vi "GetLastTrue.vi"(8 "Default value":i32, 11 "Input":bool[](array[boolean])) -> (3 "Last True":i32)   [LabVIEW 2014]
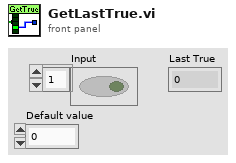
[diagram p1: front panel]
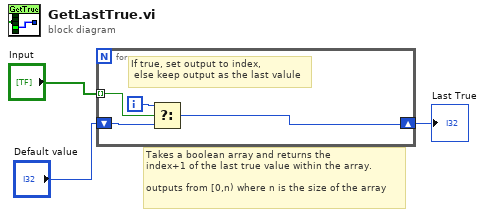
[diagram p0: block diagram]
diagram:
  # "Takes a boolean array and returns the \nindex+1 of the last true value within the array.\n\noutputs from [0,n) where n is the size of the array"
  n1 = for {
    tunnel: "Input" -> [w6] mode=indexing
    shift-right: [w7] -> w3
    shift-left: "Default value" -> [w5]
    i -> [w4]
    # "If true, set output to index,\n else keep output as the last valule"
    n2 = Select(t=w4, s=w6, f=w5) -> (s? t:f=w7:i32)
  }
  "Last True" <- w3
